vi "Check-melt-characteristics-settings.vi"(8 "error in":errorcluster, 9 "Correct. params. ref.":refnum<data-value>, 10 "Temp. params. ref.":refnum<data-value>, 11 "Analysis params. ref.":refnum<data-value>) -> (0 "error IO":errorcluster, 3 "Passed?":bool)   [LabVIEW 2013, in "CameraVision.lvlib" / "CV-Analysis.lvclass"]
uses:
  CV-Analysis.lvclass
  Temperature/CV-Temperature.lvclass
  Correction/CV-Correction.lvclass
  CV-Analysis.lvclass/CV-Analysis.ctl
  Read Melt-pool characteristics.vi
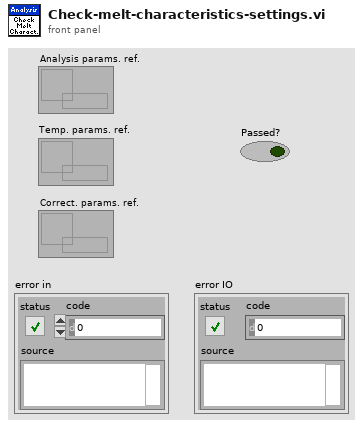
[diagram p1: front panel]
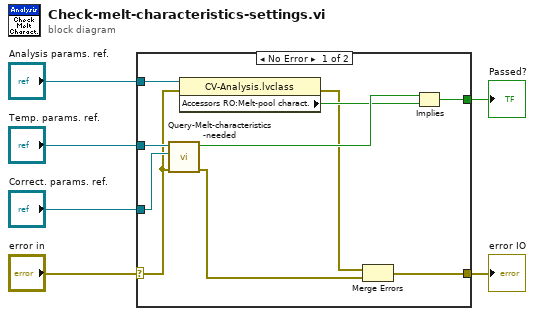
[diagram p0: block diagram]
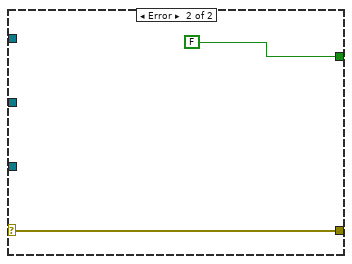
[diagram p2: hidden frame]
diagram:
  n1 = case shown="No Error" "error in" {
    selector: "error in" -> [w8 w17]
    tunnel: [w10 w17] -> w5
    tunnel: [w16 FALSE] -> w6
    tunnel: "Analysis params. ref." -> [w13 _]
    tunnel: "Temp. params. ref." -> [w14 _]
    tunnel: "Correct. params. ref." -> [w11 _]
    frame No Error {
      n2 = call "Query-Melt-characteristics-needed.vi"("error in"=w8, "Correct. params. ref."=w11, "Temp. params. ref."=w14) -> ("error IO"=w7:errorcluster, "Melt characteristics?"=w15:bool)  [unwired: 7 in]
      n3 = property class="CV-Analysis.lvclass"(reference=w13, error in=w8) -> (error out=w9:errorcluster, "Accessors RO:Melt-pool charact."=w12:bool)  [unwired: 1 out]
      n4 = Merge Errors(w9, w7) -> (w10:errorcluster)
      n5 = Implies(1:w12, 2:w15) -> (0:w16:bool)
    }
    frame Error {
    }
  }
  "Passed?" <- w6
  "error IO" <- w5
